vi "ViconN_car.vi"() -> ()   [LabVIEW 2014]
uses:
  C:/Users/Kaiyan/Desktop/Car Control PID  with vicon/ViconDataStreamSDK_DotNET.dll
  <vilib>/imath/engines/lvmath2/RunTimeEngine/Managers/WorkSpace/UID Generator.vi
  <vilib>/imath/engines/lvmath2/RunTimeEngine/BuiltInFunctions/size/NIMS_I32Row=size(GM).vi
  <vilib>/imath/engines/lvmath2/RunTimeEngine/BuiltInFunctions/max/1 input/NIMS_max(RV).vi
  <vilib>/imath/engines/lvmath2/RunTimeEngine/RangeToken/NIMS_Range_R2 - Integer.vi
  <vilib>/imath/engines/lvmath2/RunTimeEngine/IndexRead/NIMS M(S,R2).vi
  <vilib>/imath/engines/lvmath2/RunTimeEngine/BuiltInFunctions/sum/NIMS_sum(GV).vi
  <vilib>/imathl/engines/lvmath/Functions/Error Handling/Create Error.vi
  <vilib>/imath/engines/lvmath2/RunTimeEngine/IndexReplace/NIMS M(S,R2)=V.vi
  <vilib>/imath/engines/lvmath2/RunTimeEngine/ErrorHandling/NIMS_Create Error From Enums.vi
  <vilib>/imath/engines/lvmath2/RunTimeEngine/CommandStatement/MC_CommandStatement_break.vi
  <vilib>/imath/engines/lvmath2/RunTimeEngine/ArithmeticOperatorToken/NIMS_ArithmeticOperator_plus.vi
  <vilib>/imath/engines/lvmath2/RunTimeEngine/IndexRead/NIMS M(R2,S).vi
  <vilib>/imath/engines/lvmath2/RunTimeEngine/BuiltInFunctions/mean/NIMS_RS=mean(RV,I32).vi
  <vilib>/imath/engines/lvmath2/RunTimeEngine/IndexRead/NIMS M(S,S).vi
  <vilib>/imath/engines/lvmath2/RunTimeEngine/BuiltInFunctions/atan2/NIMS_atan2.vi
  <vilib>/imath/engines/lvmath2/RunTimeEngine/LocalVariableDefStatement/MC_LocalVariableDefStatement_Display.vi
  <vilib>/imath/engines/lvmath2/RunTimeEngine/RunTimeType/NIMS_RunTimeType_From StrictType (excl LVString).vi
  <vilib>/imath/engines/lvmath2/RunTimeEngine/BuiltInFunctions/length/NIMS_length(GV).vi
  <vilib>/imath/engines/lvmath2/RunTimeEngine/ArithmeticOperatorToken/NIMS_ArithmeticOperator_minus.vi
  <vilib>/imath/engines/lvmath2/RunTimeEngine/IndexRead/NIMS V(S).vi
  <vilib>/imath/engines/lvmath2/RunTimeEngine/Managers/SymbolTable/Clear UID.vi
  <vilib>/imath/engines/lvmath2/RunTimeEngine/Managers/SymbolTable/NIMS_WorkSpace.lvlib
  <vilib>/imath/engines/lvmath2/RunTimeEngine/NodeEndStatement/NIMS_NodeEndStatement_Output.vi
  <vilib>/imath/engines/lvmath2/RunTimeEngine/ErrorHandling/NIMS_Finalize Error.vi
panel:
  out "Velocity":cluster{dbl, dbl, dbl}(graph)
  out "V":dbl[](array[numeric])
  out "number":u32
  out "Ref and output ( RPM)":cluster{"initial PV":dbl, "SP:":dbl}(graph)
  out "output":dbl format="%.2f"
  in  "w_d":dbl(slide) scale=0.0..1000.0
  in  "K":dbl
  in  "K 2":dbl(slide)=0.001 scale=0.0..1.0
  out "U":dbl[](array[numeric])
  out "Sensor":dbl[](array[numeric])
  out "WheelSpeed":dbl[](array[numeric])
  out "Sampling Time 2":i32
  out "dX":dbl[](array[numeric])
  out "X":dbl[](array[numeric])
  in  "Port":u16=6340
  in  "stop 2":bool
  out "Speed":dbl[][](array[numeric])
  out "Sampling Time":i32
  in  "SubjectName":string="car_03222015"
  out "FrameRateHz":dbl
  out "FrameNumber":u32
  out "Marker Name":string[](array[string])
  in  "stop":bool
  out "MarkerCount":u32
  out "Connect Result":i32(ring) items=["Unknown", "NotImplemented", "Success", "InvalidHostName", "InvalidMulticastIP", "ClientAlreadyConnected", "ClientConnectionFailed", "ServerAlreadyTransmittingMulticast", "ServerNotTransmittingMulticast", "NotConnected", "NoFrame", "InvalidIndex", "InvalidSubjectName", "InvalidSegmentName", "InvalidMarkerName", "InvalidDeviceName", "InvalidDeviceOutputName", "InvalidLatencySampleName", "CoLinearAxes", "LeftHandedAxes", "HapticAlreadySet"]
  out "Translation":dbl[][](array[numeric])
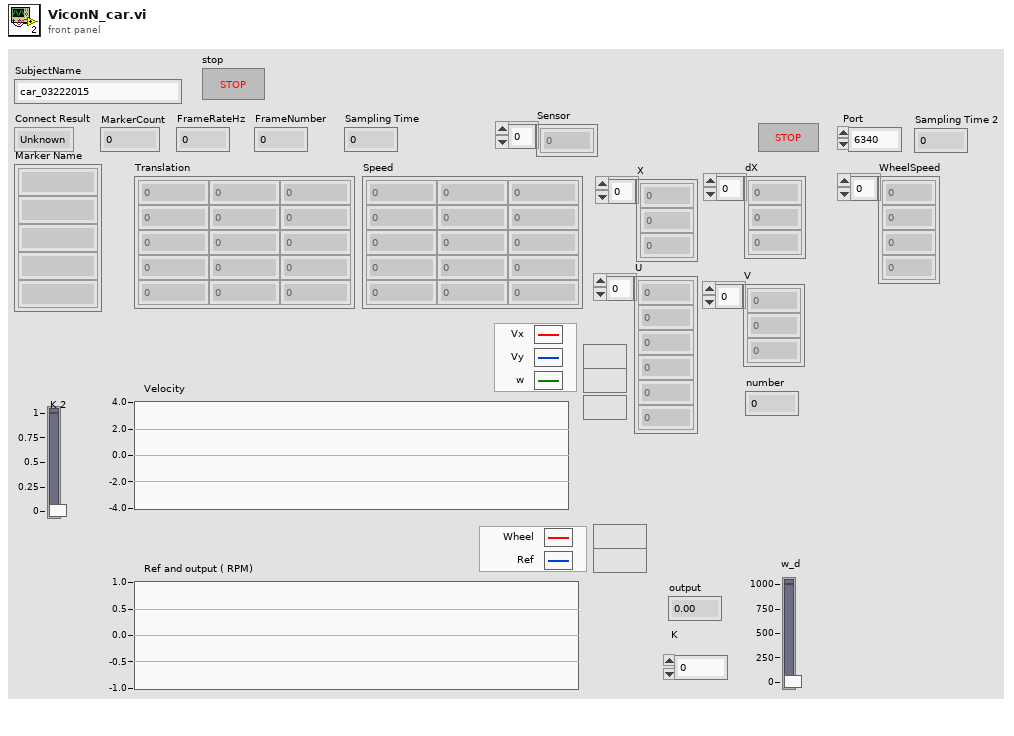
[diagram p1: front panel]
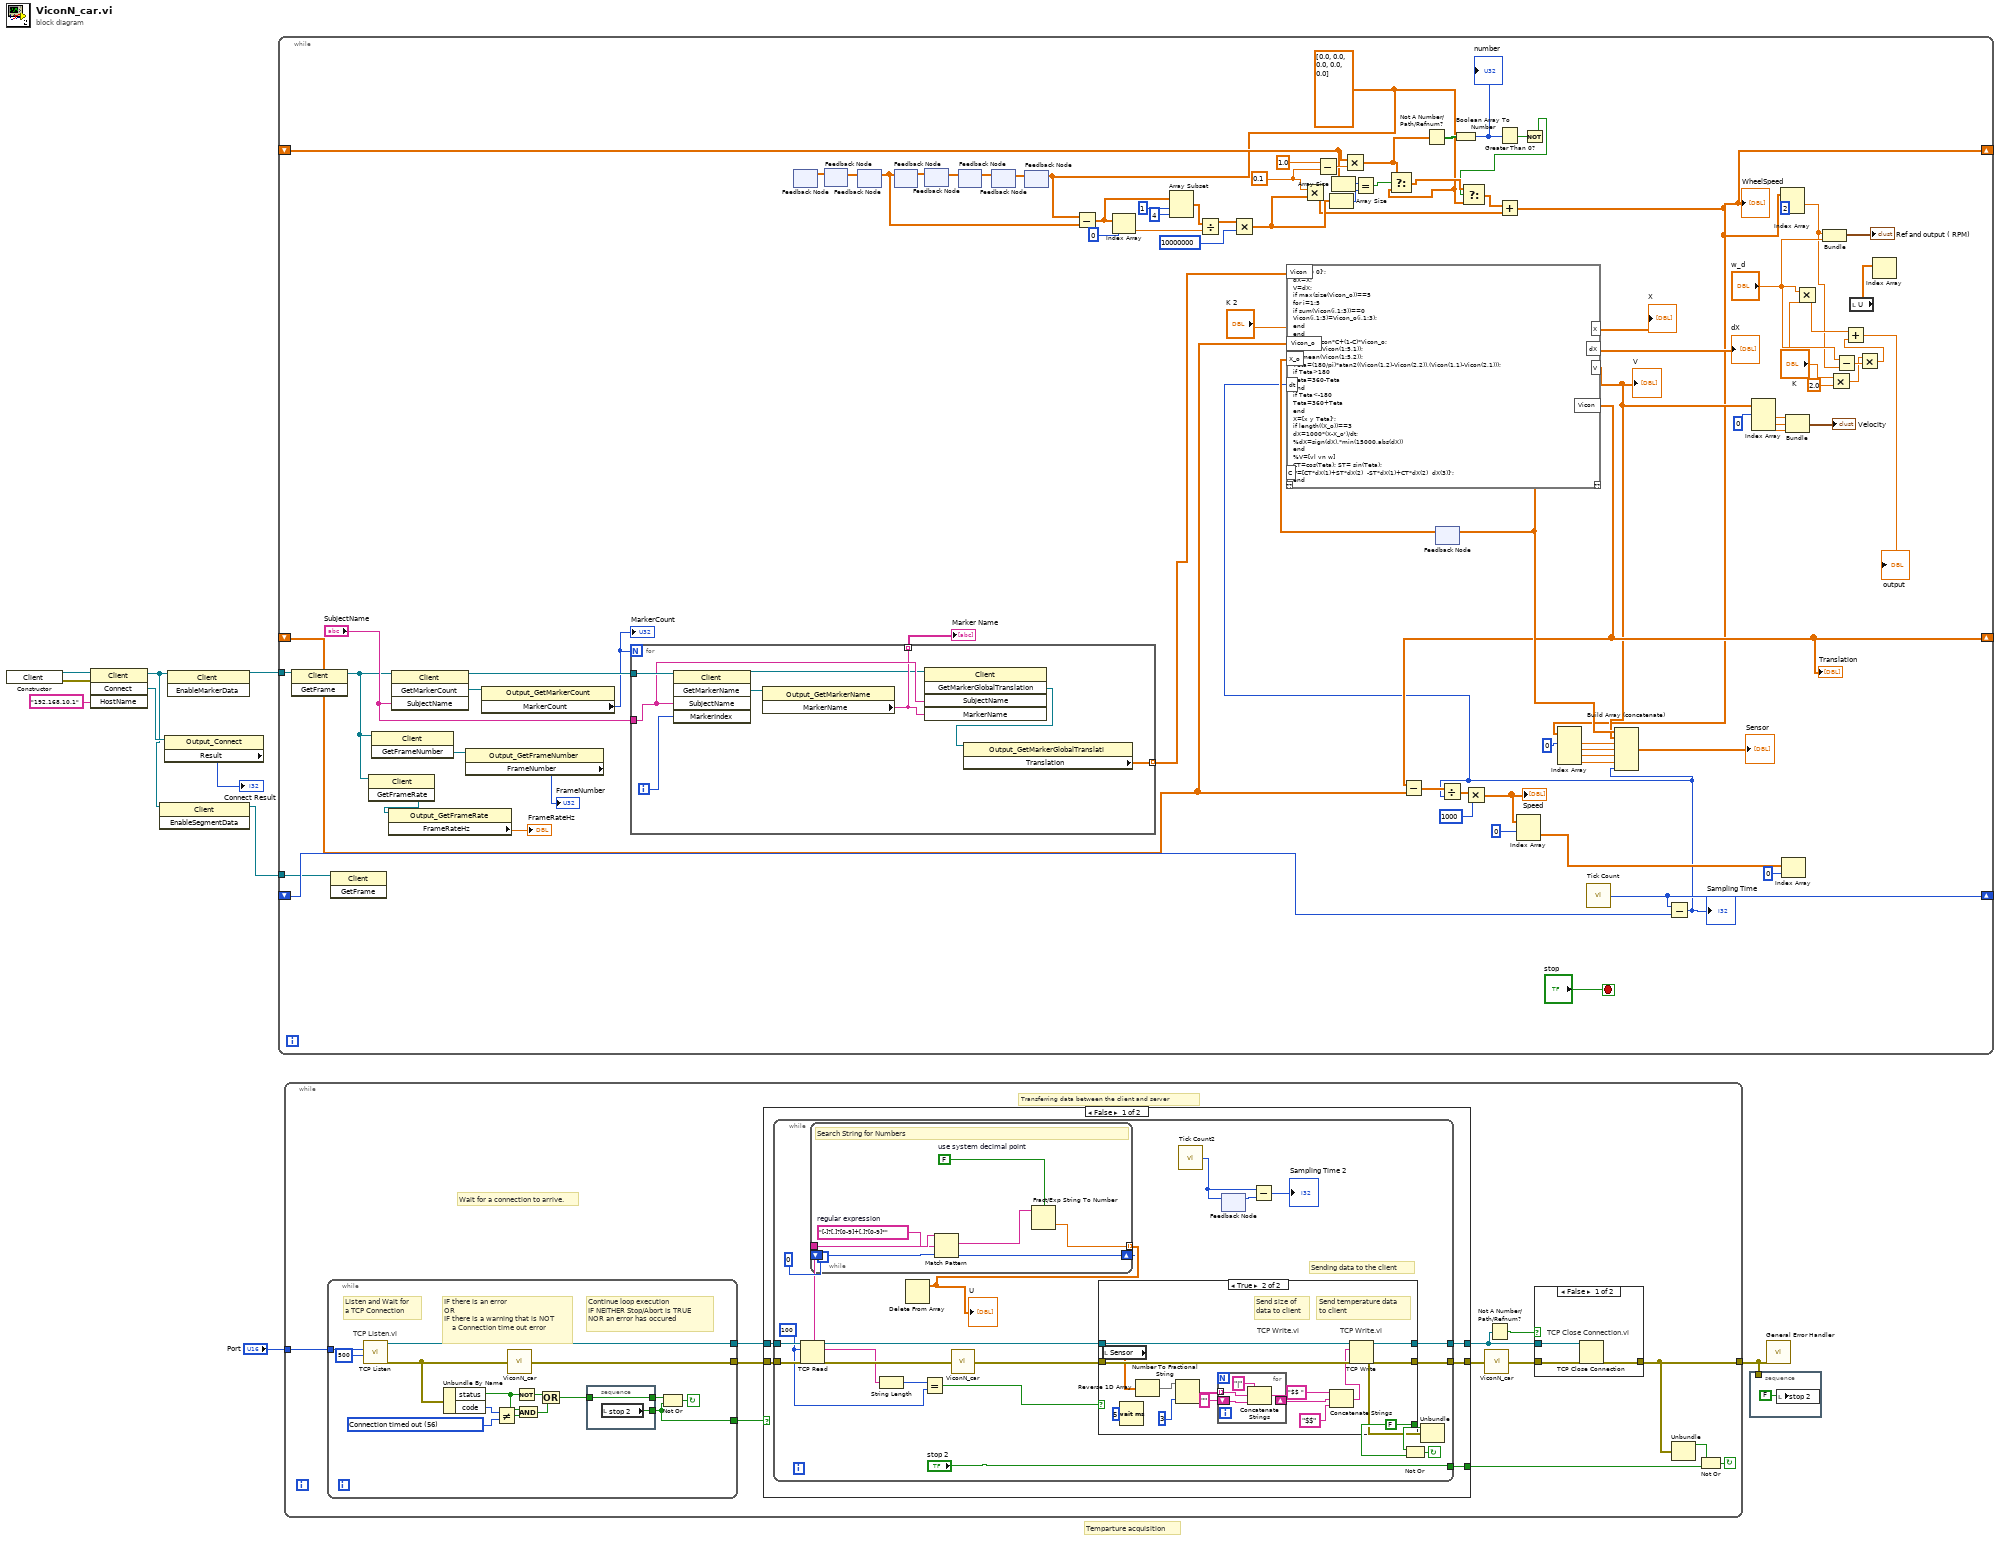
[diagram p0: block diagram]
diagram:
  # "Temparture acquisition"
  n1 = constructor class="Client"() -> (reference out=w10:refnum<k24>, error out=w9:errorcluster)  [unwired: 3 in, 1 out]
  n2 = invoke class="Client" method="Connect"(reference=w10, error in=w9, "HostName"="192.168.10.1") -> (reference out=w2:refnum<k24>, "Connect"=w7:refnum<k24>)  [unwired: 1 in, 2 out]
  n3 = invoke class="Client" method="EnableSegmentData"(reference=w2) -> (reference out=w1:refnum<k24>)  [unwired: 2 in, 2 out]
  n4 = property class="Output_Connect"(reference=w7) -> ("Result"=→"Connect Result":i32)  [unwired: 1 in, 2 out]
  n5 = invoke class="Client" method="EnableMarkerData"(reference=w2) -> (reference out=w5:refnum<k24>)  [unwired: 2 in, 2 out]
  n6 = while {
    tunnel: w5 -> [w97]
    shift-right: [w57] -> _
    shift-left: _ -> [w85]
    shift-right: [w75] -> _
    shift-left: _ -> [w79]
    shift-right: [w14] -> _
    shift-left: _ -> [w13]
    tunnel: w1 -> [w11]
    stop <- "stop" stop-if-true
    w46 = 0.1 ("K")
    w12 = dbl[] [0.0, 0.0, 0.0, 0.0, 0.0] ("f")
    n7 = invoke class="Client" method="GetFrame"(reference=w97) -> (reference out=w86:refnum<k24>)  [unwired: 2 in, 2 out]
    n8 = invoke class="Client" method="GetFrame"(reference=w11) -> ()  [unwired: 2 in, 3 out]
    n9 = invoke class="Client" method="GetFrameRate"(reference=w86) -> ("GetFrameRate"=w89:refnum<k24>)  [unwired: 2 in, 2 out]
    n10 = invoke class="Client" method="GetFrameNumber"(reference=w86) -> ("GetFrameNumber"=w91:refnum<k24>)  [unwired: 2 in, 2 out]
    n11 = property class="Output_GetFrameRate"(reference=w89) -> ("FrameRateHz"=→"FrameRateHz":dbl)  [unwired: 1 in, 2 out]
    n12 = invoke class="Client" method="GetMarkerCount"(reference=w86, "SubjectName"="SubjectName") -> (reference out=w95:refnum<k24>, "GetMarkerCount"=w96:refnum<k24>)  [unwired: 2 in, 2 out]
    n13 = property class="Output_GetFrameNumber"(reference=w91) -> ("FrameNumber"=→"FrameNumber":u32)  [unwired: 1 in, 2 out]
    n14 = property class="Output_GetMarkerCount"(reference=w96) -> ("MarkerCount"=w94:u32)  [unwired: 1 in, 2 out]
    "MarkerCount" <- w94
    n15 = for {
      N: w94 -> [_]
      tunnel: w95 -> [w594]
      tunnel: "SubjectName" -> [w592]
      tunnel: [w587] -> w76 mode=indexing
      tunnel: [w589] -> w92 mode=indexing
      i -> [w593]
      n16 = invoke class="Client" method="GetMarkerName"(reference=w594, "SubjectName"=w592, "MarkerIndex"=w593) -> (reference out=w588:refnum<k24>, "GetMarkerName"=w591:refnum<k24>)  [unwired: 2 in, 3 out]
      n17 = property class="Output_GetMarkerName"(reference=w591) -> ("MarkerName"=w589:string)  [unwired: 1 in, 2 out]
      n18 = invoke class="Client" method="GetMarkerGlobalTranslation"(reference=w588, "SubjectName"=w592, "MarkerName"=w589) -> ("GetMarkerGlobalTranslation"=w590:refnum<k24>)  [unwired: 2 in, 4 out]
      n19 = property class="Output_GetMarkerGlobalTranslati"(reference=w590) -> ("Translation"=w587:dbl[])  [unwired: 1 in, 2 out]
    }
    "Marker Name" <- w92
    n20 = feedback #1() -> ()  [unwired: 2 in]
    n21 = feedback #2() -> (w64:dbl[])  [unwired: 1 in]
    n22 = feedback-in #1(w64) -> ()
    n23 = feedback #3() -> (w65:dbl[])  [unwired: 1 in]
    n24 = feedback-in #2(w65) -> ()
    n25 = feedback #4() -> (w32:dbl[])  [unwired: 1 in]
    n26 = feedback-in #3(w32) -> ()
    n27 = feedback #5() -> (w66:dbl[])  [unwired: 1 in]
    n28 = feedback-in #4(w66) -> ()
    n29 = feedback #6() -> (w73:dbl[])  [unwired: 1 in]
    n30 = feedback-in #5(w73) -> ()
    n31 = feedback #7() -> (w74:dbl[])  [unwired: 1 in]
    n32 = feedback-in #6(w74) -> ()
    n33 = feedback-in #8(w12) -> ()
    n34 = feedback #8() -> (w42:dbl[])  [unwired: 1 in]
    n35 = feedback-in #7(w42) -> ()
    n36 = Subtract(x=w12, y=w32) -> (x-y=w67:dbl[])
    n37 = Index Array(array=w67, index=0 ("index (row)")) -> (element=w71:dbl)
    n38 = Array Subset(array=w67, index=1 ("index (row)"), length=4 ("index (row)")) -> (w68:dbl[])
    n39 = Divide(x=w68, y=w71) -> (x/y=w62:dbl[])
    n40 = Multiply(x=w62, y=10000000 ("index (row)")) -> (x*y=w44:dbl[])
    n41 = Multiply(x=w46, y=w44) -> (x*y=w43:dbl[])
    n42 = Subtract(x=1.0, y=w46) -> (x-y=w50:dbl)
    n43 = Array Size(array=w44) -> (size(s)=w47:i32)
    n44 = Array Size(array=w13) -> (size(s)=w49:i32)
    n45 = Multiply(x=w13, y=w50) -> (x*y=w36:dbl[])
    n46 = Equal?(x=w49, y=w47) -> (x = y?=w48:bool)
    n47 = Select(t=w36, s=w48, f=w12) -> (s? t:f=w37:dbl[])
    n48 = Not A Number/Path/Refnum?(number/path/refnum=w36) -> (NaN/Path/Refnum?=w41:bool[])
    n49 = feedback #9() -> (w78:dbl[])  [unwired: 1 in]
    n50 = Boolean Array To Number(Boolean array=w41) -> (number=w40:u32)
    "number" <- w40
    n51 = Greater Than 0?(x=w40) -> (x > 0?=w39:bool)
    n52 = Not(x=w39) -> (.not. x?=w35:bool)
    n53 = Select(t=w37, s=w35, f=w12) -> (s? t:f=w38:dbl[])
    n54 = Add(x=w38, y=w43) -> (x+y=w14:dbl[])
    "WheelSpeed" <- w14
    n55 = Index Array(array=w14, index #1=0 ("index (row)")) -> (element #1=w56:dbl, element #2=w55:dbl, element #3=w54:dbl, element #4=w53:dbl)  [unwired: 3 in]
    n56 = call "Tick Count"() -> ("Tick Count(mSec)"=w57:u32)
    n57 = Subtract(x=w57, y=w85) -> (x-y=w51:u32)
    "Sampling Time" <- w51
    n58 = mathscript code="X=[0 0 0]';\ndX=X;\nV=dX;\nif max(size(Vicon_o))==5\nfor i=1:5\nif sum(Vicon(i,1:3))==0\nVicon(i,1:3)=Vicon_o(i,1:3);\nend\nend\nVicon=Vicon*C+(1-C)*Vicon_o;\nx=mean(Vicon(1:5,1));\ny=mean(Vicon(1:5,2));\nTeta=(180/pi)*atan2((Vicon(1,2)-Vicon(2,2)),(Vicon(1,1)-Vicon(2,1)));\nif Teta>180\nTeta=360-Teta\nend\nif Teta<-180\nTeta=360+Teta\nend\nX=[x y Teta]';\nif length((X_o))==3\ndX=1000*(X-X_o')/dt;\n%dX=sign(dX).*min(15000,abs(dX))\nend\n%V=[vl vn w]\nCT=cos(Teta); ST= sin(Teta);\nV=[CT*dX(1)+ST*dX(2)  -ST*dX(1)+CT*dX(2)  dX(3)]';\nend"("Vicon"=w76, "Vicon_o"=w79, "C"="K 2", "X_o"=w78, "dt"=w51) -> ("Vicon"=w75:dbl[][], "X"=w77:dbl[], "dX"=→"dX":dbl[], "V"=w15:dbl[])  [unwired: 1 in, 1 out]
    "Translation" <- w75
    "X" <- w77
    "V" <- w15
    n59 = Subtract(x=w75, y=w79) -> (x-y=w84:dbl[][])
    n60 = feedback-in #9(w77) -> ()
    n61 = Divide(x=w84, y=w51) -> (x/y=w83:dbl[][])
    n62 = Multiply(x=w83, y=1000 ("index (row)")) -> (x*y=w81:dbl[][])
    "Speed" <- w81
    n63 = Index Array(array=w81, index (row)=0) -> (element=w59:dbl[])  [unwired: 1 in]
    n64 = Build Array (concatenate)(w77, w15, w56, w55, w54, w53, w51) -> (→"Sensor":dbl[])
    n65 = Index Array(array=w15, index #1=0 ("index")) -> (element #1=w19:dbl, element #2=w18:dbl, element #3=w17:dbl)  [unwired: 2 in]
    n66 = Index Array(array=w14, index #1=2 ("index")) -> (element #1=w26:dbl)  [unwired: 1 in, 1 out]
    n67 = Index Array(array=w59, index=0 ("index (row)")) -> ()  [unwired: 1 out]
    n68 = Bundle(w19, w18, w17) -> (→"Velocity":cluster{dbl, dbl, dbl})  [unwired: 1 in]
    n69 = Multiply(x="w_d", y="K") -> (x*y=w30:dbl)
    n70 = Bundle(w26, "w_d"="w_d") -> (→"Ref and output ( RPM)":cluster{dbl, "w_d":dbl})  [unwired: 1 in]
    n71 = Multiply(x="K", y=2.0) -> (x*y=w22:dbl)
    n72 = Subtract(x="w_d", y=w26) -> (x-y=w25:dbl)
    n73 = local read "U"() -> (w28:dbl[])
    n74 = Multiply(x=w22, y=w25) -> (x*y=w24:dbl)
    n75 = Add(x=w30, y=w24) -> (x+y=→"output":dbl)
    n76 = Index Array(array=w28) -> ()  [unwired: 1 in, 1 out]
  }
  n77 = while {
    tunnel: "Port" -> [w604]
    tunnel: [w600] -> w4
    stop <- w605 continue-if-true
    # "Transferring data between the client and server"
    # "Wait for a connection to arrive."
    n78 = while {
      tunnel: w604 -> [w683]
      tunnel: [w682] -> w603
      tunnel: [w673] -> w602
      tunnel: [w674] -> w598
      stop <- w679 continue-if-true
      w672 = u16 56 items=["No Error", "Argument Error", "Memory Full", "Out of Zone", "End of File", "File Already Open", "Generic File IO Error", "File Not Found", "File Permission Error", "Disk Full", "Duplicate Path", "Too Many Files Open", "Not Enabled", "Resource File Not Found", "Cannot Add Resource", "Resource Not Found", "Image Not Found", "Image Memory Error", "Pen Does Not Exist", "Config Bad Type", "Config Token Not Found", "Config Parse Error", "Config Memory Error", "Bad External Code Format", "Bad External Code Offset", "External Code Not Present", "Null Window", "Destroy Window Mixup", "Null Menu", "Print Aborted", "Bad Print Record", "Print Driver Error", "Windows Error During Print", "Memory Error During Print", "Print Dialog Error", "Generic Print Error", "Invalid Device Refnum", "Device Not Found", "Device Parameter Error", "Device Unit Error", "Can't Open Device", "Device Call Aborted", "Generic Error", "Cancelled By User", "Object ID Too Low", "Object ID Too High", "Object Not In Heap", "Unknown Heap", "Bad DefProc ID", "DefProc Not In Table", "Message Out Of Range", "Null Method", "Unknown Message", "Manager Call Not Supported", "Bad address", "Connection In progress", "Connection timed out", "Connection is already in progress", "Network attribute not supported", "Network error", "Address in use", "System out of memory", "Connection aborted", "Connection refused", "Connection is not connected", "Connection is already connected", "Connection closed", "Initialize error (interapplication manager)", "Bad occurrence", "Wait on unbound occurrence handler", "Occurrence queue overflow", "Bad path", "Semaphore not signaled", "Unrecognized type (interapplication manager)"]
      # "Listen and Wait for\na TCP Connection"
      # "Continue loop execution\nIF NEITHER Stop/Abort is TRUE\nNOR an error has occured"
      # "IF there is an error \nOR\nIF there is a warning that is NOT\n    a Connection time out error"
      # "TCP Listen.vi"
      n79 = call <vilib>:"TCP Listen.vi"("timeout ms (wait forever: -1)"=500, "port"=w683) -> ("error out"=w671:errorcluster, "connection ID"=w682:refnum<k5>)  [unwired: 5 in, 3 out]
      n80 = Unbundle By Name(w671) -> ("status"=w670:bool, "code"=w669:i32)
      n81 = Not Equal?(x=w669, y=w672) -> (x != y?=w680:bool)
      n82 = call "ViconN_car.vi"("error in (no error)"=w671) -> ("error out"=w673:errorcluster)  [unwired: 14 in]
      n83 = Not(x=w670) -> (.not. x?=w678:bool)
      n84 = And(x=w670, y=w680) -> (x .and. y?=w677:bool)
      n85 = Or(x=w678, y=w677) -> (x .or. y?=w676:bool)
      n86 = stacked-sequence {
        tunnel: w676 -> [w685]
        tunnel: [w685] -> w675
        tunnel: [w684] -> w674
        frame #0 {
          n87 = local read "stop 2"() -> (w684:bool)
        }
      }
      n88 = Not Or(1:w674, 2:w675) -> (0:w679:bool)
    }
    n89 = case shown="False" w598 {
      selector: w598 -> [_ w662]
      tunnel: [w611 w663] -> w606
      tunnel: w603 -> [w610 w664]
      tunnel: w602 -> [w609 w663]
      tunnel: [w608 w664] -> w597
      tunnel: [w607 w662] -> w595
      frame False {
        n90 = while {
          tunnel: w610 -> [w628]
          tunnel: [w625] -> w608
          tunnel: [w623] -> w611
          tunnel: w609 -> [w629]
          tunnel: ["stop 2"] -> w607
          stop <- w630 continue-if-true
          w619 = 100
          # "Sending data to the client"
          n91 = TCP Read(connection ID=w628, bytes to read=w619, error in (no error)=w629) -> (connection ID out=w626:refnum<k5>, data out=w616:string, error out=w627:errorcluster)  [unwired: 2 in]
          n92 = while {
            tunnel: w616 -> [w639]
            shift-left: 0 -> [w636]
            shift-right: [w634] -> _
            tunnel: [w638] -> w612 mode=indexing
            stop <- w637 stop-if-true
            w635 = FALSE  # use system decimal point
            w633 = "[-]?[.]?[0-9]+[.]?[0-9]*"  # regular expression
            # "Search String for Numbers"
            n93 = Match Pattern(string=w639, regular expression=w633, offset (0)=w636) -> (match substring=w632:string, offset past match=w634:i32)  [unwired: 2 out]
            n94 = Fract/Exp String To Number(use system decimal point (T)=w635, string=w632) -> (number=w638:dbl)  [unwired: 2 in, 1 out]
            n95 = Less Than 0?(x=w634) -> (x < 0?=w637:bool)
          }
          "U" <- w612
          n96 = String Length(string=w616) -> (length=w620:i32)
          n97 = Delete From Array(array=w612) -> ()  [unwired: 2 in, 2 out]
          n98 = Equal?(x=w620, y=w619) -> (x = y?=w618:bool)
          n99 = call "ViconN_car.vi"("error in (no error)"=w627) -> ("error out"=w622:errorcluster)  [unwired: 14 in]
          n100 = case shown="True" w618 {
            tunnel: w622 -> [w641 w653]
            tunnel: w626 -> [w640 w654]
            tunnel: [w640 w657] -> w625
            tunnel: [w641 w656] -> w623
            tunnel: [TRUE FALSE] -> w624
            frame False {
              # "Wait for Client to read all sent data"
            }
            frame True {
              # "Send temperature data\nto client"
              # "Send size of \ndata to client"
              # "TCP Write.vi"
              # "TCP Write.vi"
              n101 = local read "Sensor"() -> (w643:dbl[])
              n102 = Wait (ms)(milliseconds to wait=u32 5) -> ()  [unwired: 1 out]
              n103 = Reverse 1D Array(array=w643) -> (reversed array=w645:dbl[])
              n104 = Number To Fractional String(number=w645, precision (6)=u32 3 ("milliseconds to wait")) -> (F-format string=w651:string[])  [unwired: 2 in]
              n105 = for {
                tunnel: w651 -> [w661] mode=indexing
                shift-right: [w659] -> w646
                shift-left: "" -> [w660]
                n106 = Concatenate Strings("|", w661, w660) -> (w659:string)
              }
              n107 = Concatenate Strings("$$ ", w646, "$$") -> (w648:string)
              n108 = TCP Write(connection ID=w654, data in=w648, error in (no error)=w653) -> (connection ID out=w657:refnum<k5>, error out=w656:errorcluster)  [unwired: 1 in, 1 out]
            }
          }
          n109 = call "Tick Count2"() -> ("Tick Count(mSec)"=w614:u32)
          n110 = feedback-in #10(w614) -> ()
          n111 = feedback #10() -> (w613:u32)  [unwired: 1 in]
          n112 = Subtract(x=w614, y=w613) -> (x-y=→"Sampling Time 2":u32)
          n113 = Unbundle(w623) -> ("status"=w631:bool)  [unwired: 2 out]
          n114 = Not Or(1:w624, 2:w631) -> (0:w630:bool)
        }
      }
      frame True {
      }
    }
    n115 = call "ViconN_car.vi"("error in (no error)"=w606) -> ("error out"=w599:errorcluster)  [unwired: 4 in]
    n116 = Not A Number/Path/Refnum?(number/path/refnum=w597) -> (NaN/Path/Refnum?=w596:bool)
    n117 = case shown="False" w596 {
      tunnel: w599 -> [w667 w668]
      tunnel: w597 -> [w666 _]
      tunnel: [w665 w668] -> w600
      frame False {
        # "TCP Close Connection.vi"
        n118 = TCP Close Connection(connection ID=w666, error in (no error)=w667) -> (error out=w665:errorcluster)  [unwired: 1 in, 1 out]
      }
      frame True {
      }
    }
    n119 = Unbundle(w600) -> ("status"=w601:bool)  [unwired: 2 out]
    n120 = Not Or(1:w595, 2:w601) -> (0:w605:bool)
  }
  n121 = stacked-sequence {
    tunnel: w4 -> [_]
    frame #0 {
      n122 = local write "stop 2"(FALSE) -> ()
    }
  }
  n123 = call <vilib>:"General Error Handler.vi"("error in (no error)"=w4) -> ()  [unwired: 10 in, 5 out]
